vi "修改探头名称.vi"(9 "探头信息":string[](array[string]), 10 "原名称":string, 11 "输入信息":string) -> (0 "确定修改？":bool, 3 "新名称 o":string caption="新备注")   [LabVIEW 2017]
uses:
  <vilib>/addons/database/NI_Database_API.lvlib
panel:
  out "非空提示":string caption="字符串"
  in  "新名称":string caption="新备注"
  in  "取消":bool
  in  "确定":bool caption="OK2"
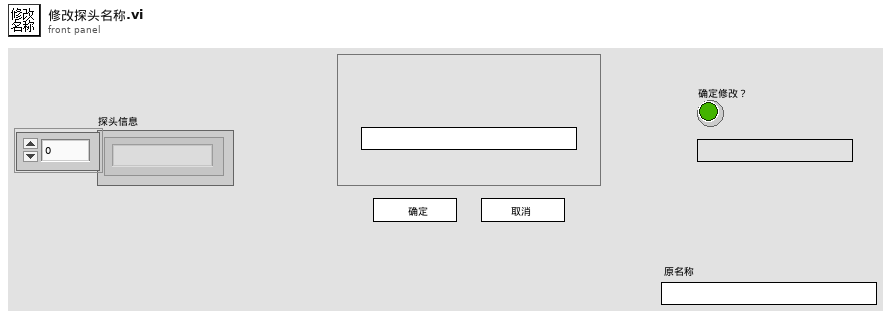
[diagram p1: front panel]
types:
  T1 = enum32{"Invalid", "Standard", "Closed", "Hidden", "Minimized", "Maximized"}
  T2 = cluster{"设备名称":string, "启用累积？":bool, "起始时间":timestamp, "累积剂量":dbl, "累积报警阈值":dbl}
  T3 = typedef "NI_Database_API.lvlib/Conn ObjectReference.ctl" = refnum<k1>
  T4 = cluster{"设备名称":string, "启用累积？":bool, "起始时间":timestamp, "累积剂量":dbl, "累积报警阈值":dbl}[]
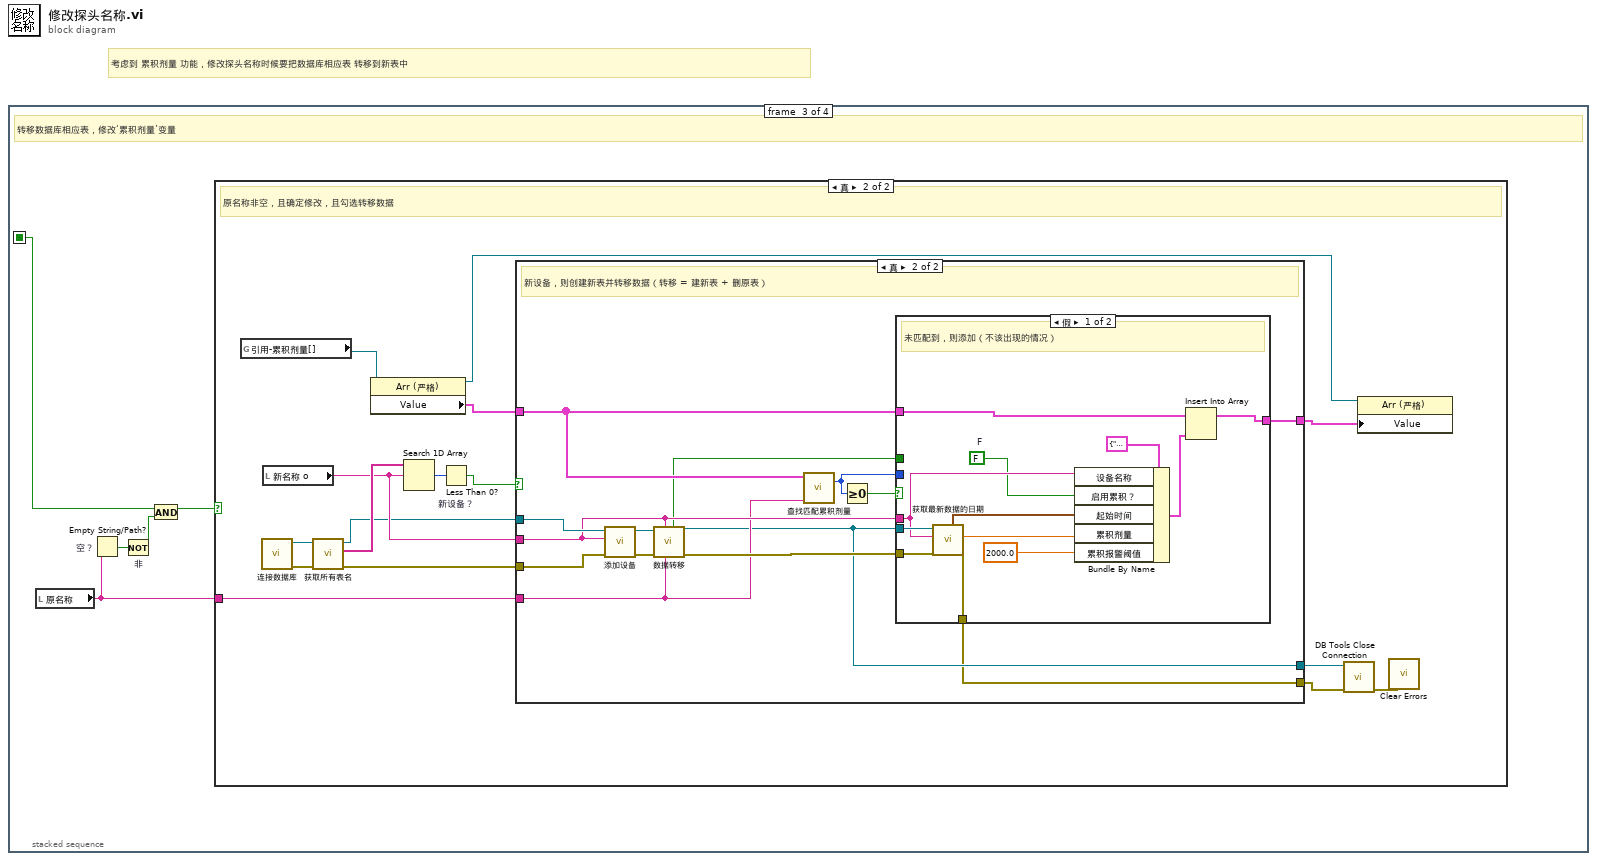
[diagram p0: block diagram]
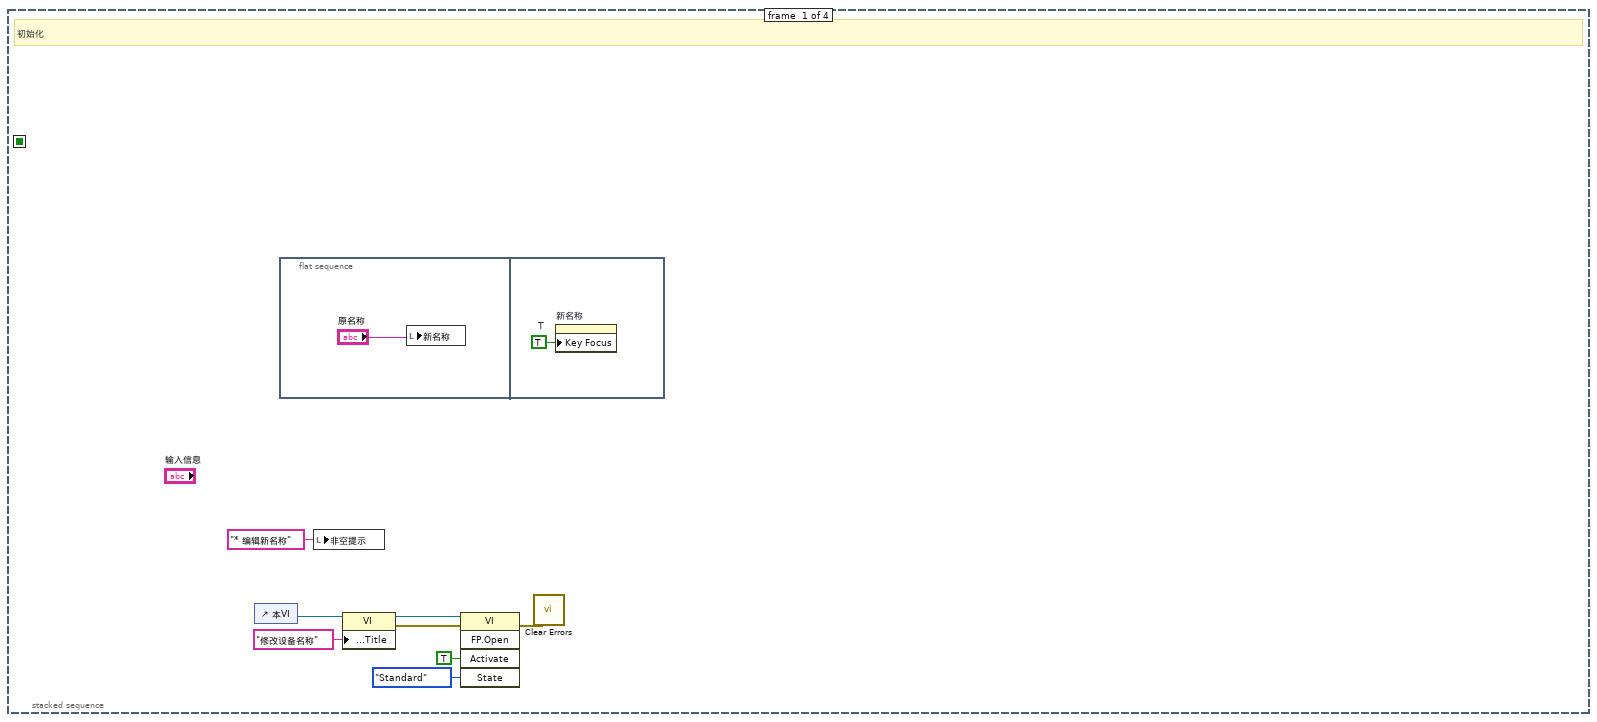
[diagram p2: hidden frame]
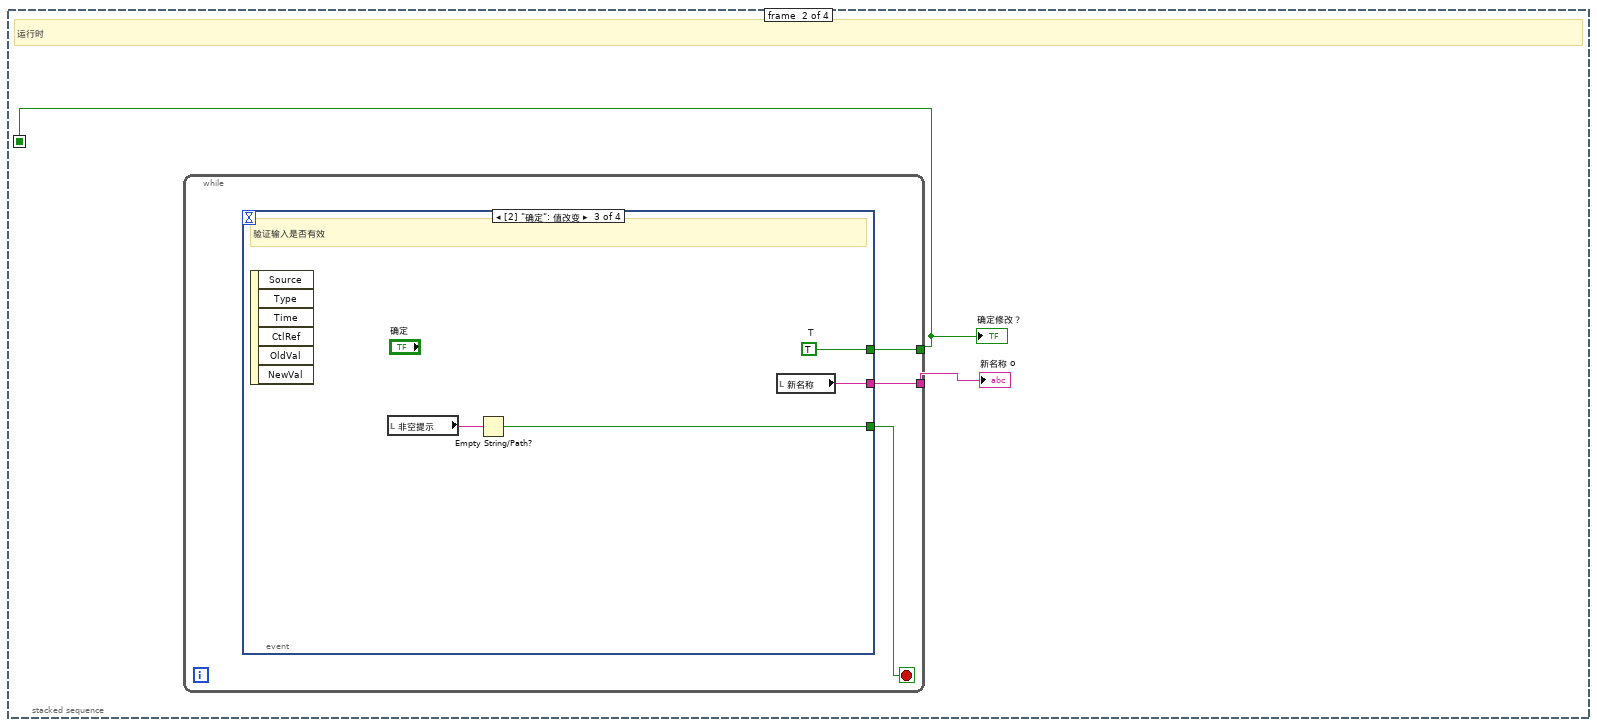
[diagram p3: hidden frame]
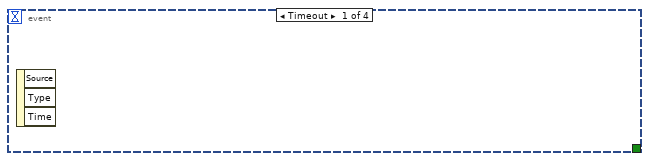
[diagram p4: hidden frame]
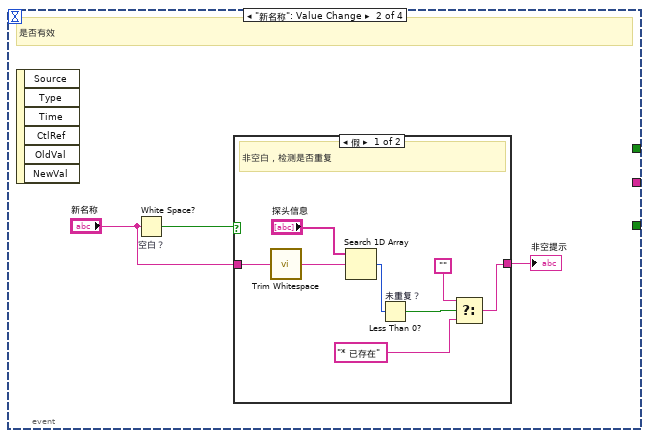
[diagram p5: hidden frame]
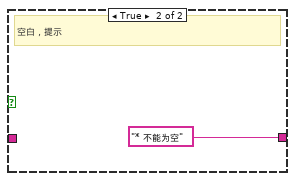
[diagram p6: hidden frame]
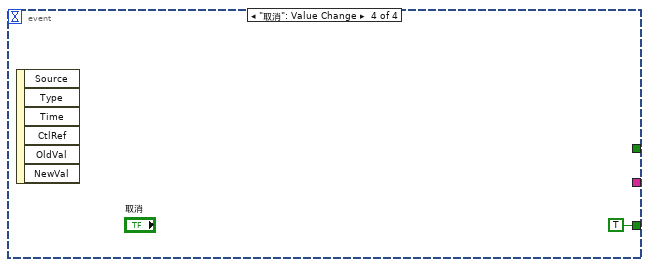
[diagram p7: hidden frame]
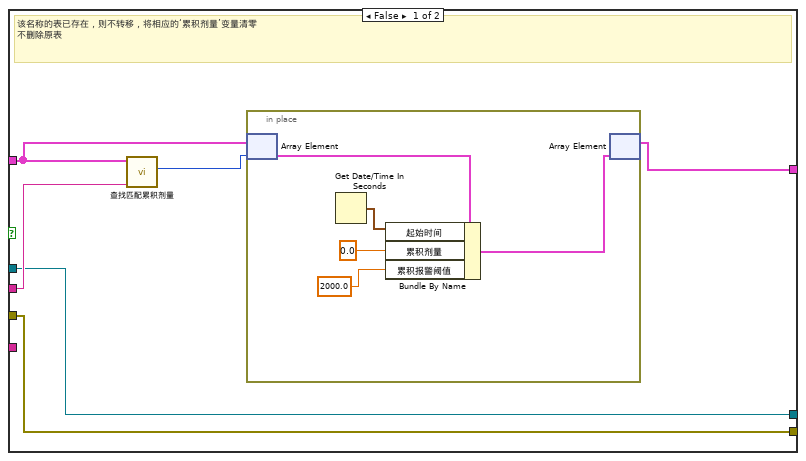
[diagram p9: hidden frame]
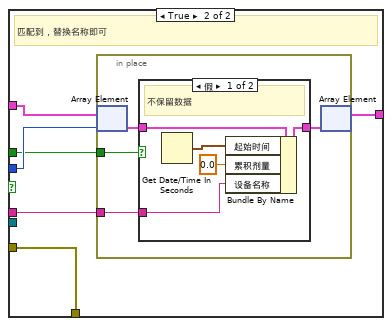
[diagram p10: hidden frame]
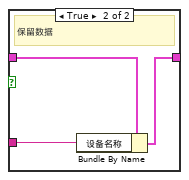
[diagram p11: hidden frame]
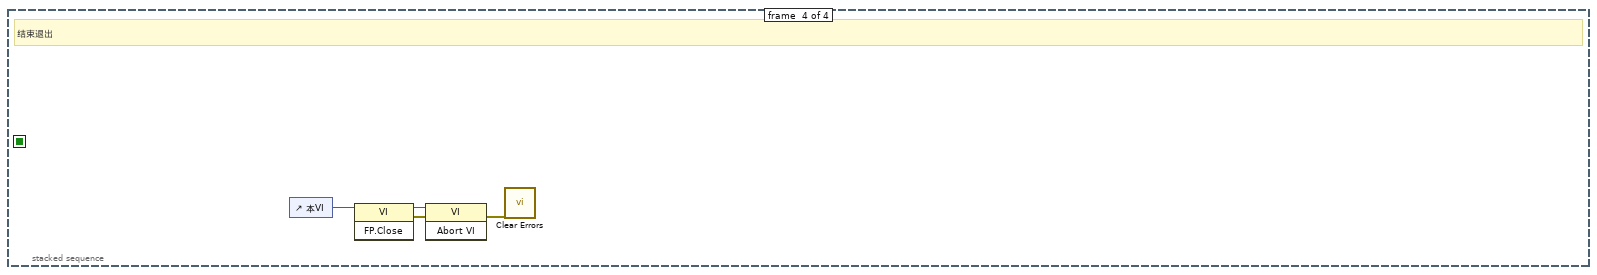
[diagram p12: hidden frame]
diagram:
  # "考虑到 累积剂量 功能，修改探头名称时候要把数据库相应表 转移到新表中"
  n1 = stacked-sequence {
    seq-local: [_ w11 _ _] -> [_ _ w37 _]
    frame #0 {
      # "初始化"
      n2 = control-ref of="本VI"() -> (w6:refnum<vi>)
      n3 = flat-sequence {
        frame #0 {
          n4 = local write "新名称"("原名称") -> ()
        }
        frame #1 {
          w10 = TRUE  # T
          n5 = property on="新名称" class="Str"("Key Focus"=w10) -> ()  [unwired: 2 in, 2 out]
        }
      }
      n6 = local write "非空提示"("* 编辑新名称" ("非空提示")) -> ()
      n7 = property class="VI"(reference=w6, "Front Panel.Title"="修改设备名称" ("前面板窗口:标题")) -> (reference out=w5:refnum<vi>, error out=w2:errorcluster)  [unwired: 1 in]
      n8 = invoke class="VI" method="FP.Open"(reference=w5, error in=w2, "Activate"=TRUE ("激活？"), "State"=T1."Standard" ("状态")) -> (error out=w1:errorcluster)  [unwired: 1 in, 4 out]
      n9 = call <vilib>:"Clear Errors.vi"("error in (no error)"=w1) -> ()  [unwired: 5 in, 2 out]
    }
    frame #1 {
      # "运行时"
      n10 = while {
        tunnel: [w14] -> w11
        tunnel: [w13] -> w12
        stop <- w15 stop-if-true
        n11 = event shown="[2] \"确定\": 值改变" {
          selector: _ -> [_ _ _ _]
          dyn-events: _ -> [_ _ _ _]
          timeout: _ -> [_ _ _ _]
          tunnel: [_ _ w30 TRUE] -> w15
          tunnel: [_ _ w29 _] -> w14
          tunnel: [_ _ w28 _] -> w13
          event Timeout {
            n12 = event-data() -> ()  [unwired: 1 in, 3 out]
          }
          event "新名称": Value Change {
            # "是否有效"
            n13 = event-data() -> ()  [unwired: 1 in, 6 out]
            n14 = White Space? "空白？"(1:"新名称") -> (0:w18:bool)
            n15 = case shown="假" w18 {
              tunnel: [w19 "* 不能为空" ("非空提示")] -> w17
              tunnel: "新名称" -> [w25 _]
              frame False {
                # "非空白，检测是否重复"
                n16 = call <vilib>:"Trim Whitespace.vi"("string"=w25) -> ("trimmed string"=w24:string)  [unwired: 1 in]
                n17 = Search 1D Array(1D array="探头信息", element=w24) -> (index of element=w23:i32)  [unwired: 1 in]
                n18 = Less Than 0? "未重复？"(x=w23) -> (x < 0?=w22:bool)
                n19 = Select(t="", s=w22, f="* 已存在") -> (s? t:f=w19:string)
              }
              frame True {
                # "空白，提示"
              }
            }
            "非空提示" <- w17
          }
          event "确定": Value Change {
            w29 = TRUE  # T
            # "验证输入是否有效"
            n20 = event-data() -> ()  [unwired: 1 in, 6 out]
            n21 = local read "非空提示"() -> (w31:string)
            n22 = Empty String/Path?(string/path=w31) -> (empty?=w30:bool)
            n23 = local read "新名称"() -> (w28:string)
          }
          event "取消": Value Change {
            n24 = event-data() -> ()  [unwired: 1 in, 6 out]
          }
        }
      }
      "新名称 o" <- w12
      "确定修改？" <- w11
    }
    frame #2 {
      # "转移数据库相应表，修改‘累积剂量’变量"
      n25 = local read "原名称"() -> (w36:string)
      n26 = Empty String/Path? "空？"(string/path=w36) -> (empty?=w35:bool)
      n27 = Not "非"(x=w35) -> (.not. x?=w33:bool)
      n28 = And(x=w37, y=w33) -> (x .and. y?=w34:bool)
      n29 = case shown="真" w34 {
        tunnel: w36 -> [_ w41]
        frame False {
          # "取消修改"
        }
        frame True {
          # "原名称非空，且确定修改，且勾选转移数据"
          n30 = global read "全局变量-35点监测.vi" "引用-累积剂量[]"() -> (w45:refnum<vi>)
          n31 = call "连接数据库.vi"() -> ("error out"=w53:errorcluster, "connection reference"=w52:T3)  [unwired: 10 in]
          n32 = local read "新名称 o"() -> (w48:string)
          n33 = call "获取所有表名.vi"("error in (no error)"=w53, "数据库连接引用 i"=w52) -> ("error out"=w47:errorcluster, "表名"=w51:string[], "数据库连接引用 o"=w46:T3)  [unwired: 7 in]
          n34 = property class="Arr (严格)"(reference=w45) -> (reference out=w43:refnum<vi>, "Value"=w44:T4)  [unwired: 1 in, 1 out]
          n35 = Search 1D Array(1D array=w51, element=w48) -> (index of element=w50:i32)  [unwired: 1 in]
          n36 = Less Than 0? "新设备？"(x=w50) -> (x < 0?=w49:bool)
          n37 = case shown="真" w49 {
            tunnel: w48 -> [w59 w72]
            tunnel: w47 -> [w54 w76]
            tunnel: w46 -> [w55 w75]
            tunnel: [w56 w71] -> w42
            tunnel: w41 -> [_ w69]
            tunnel: w44 -> [w58 w68]
            tunnel: [w55 w67] -> w40
            tunnel: [w54 w66] -> w39
            frame False {
              # "该名称的表已存在，则不转移，将相应的‘累积剂量’变量清零\n不删除原表"
              n38 = call "查找匹配累积剂量.vi"("探头名称"=w59, "累积剂量"=w58) -> ("匹配索引"=w57:i32)  [unwired: 7 in, 2 out]
              n39 = in-place {
                n40 = in-place-array #1(w58, w57) -> (w64:T2)
                n41 = Get Date/Time In Seconds() -> (seconds since 1Jan1904=w62:timestamp)
                n42 = Bundle By Name(cluster=w64, "起始时间"=w62, "累积剂量"=0.0, "累积报警阈值"=2000.0 ("累积剂量")) -> (w63:T2)
                n43 = in-place-array #1(w63) -> (w56:T4)  [unwired: 1 out]
              }
            }
            frame True {
              # "新设备，则创建新表并转移数据（转移 = 建新表 + 删原表）"
              n44 = call "添加设备.vi"("error in (no error)"=w76, "设备名称"=w72, "数据库连接引用 i"=w75) -> ("error out"=w77:errorcluster, "数据库连接引用 o"=w78:T3)  [unwired: 7 in]
              n45 = call "数据转移.vi"("原表名"=w69, "新表名"=w72, "error in (no error)"=w77, "数据库连接引用 i"=w78) -> ("error out"=w70:errorcluster, "数据库连接引用 o"=w67:T3, "保留数据？"=w65:bool)  [unwired: 5 in]
              n46 = call "查找匹配累积剂量.vi"("探头名称"=w69, "累积剂量"=w68) -> ("匹配索引"=w73:i32)  [unwired: 7 in, 2 out]
              n47 = Greater Or Equal To 0?(x=w73) -> (x >= 0?=w74:bool)
              n48 = case shown="假" w74 {
                tunnel: w73 -> [_ w95]
                tunnel: w68 -> [w88 w96]
                tunnel: w72 -> [w86 w94]
                tunnel: [w80 w93] -> w71
                tunnel: w67 -> [w90 _]
                tunnel: w70 -> [w89 w92]
                tunnel: [w79 w92] -> w66
                tunnel: w65 -> [_ w91]
                frame False {
                  w85 = FALSE  # F
                  # "未匹配到，则添加（不该出现的情况）"
                  n49 = call "获取最新数据的日期.vi"("error in (no error)"=w89, "表名"=w86, "数据库连接引用 i"=w90) -> ("error out"=w79:errorcluster, "累积值"=w83:dbl, "起始时间"=w84:timestamp)  [unwired: 4 in, 2 out]
                  n50 = Bundle By Name(cluster=T2 {"设备名称"="", "启用累积？"=FALSE, "起始时间"=timestamp(0 s since 1904-01-01), "累积剂量"=0.0, "累积报警阈值"=0.0} ("累积剂量"), "设备名称"=w86, "启用累积？"=w85, "起始时间"=w84, "累积剂量"=w83, "累积报警阈值"=2000.0) -> (w81:T2)
                  n51 = Insert Into Array(array=w88, new element=w81) -> (w80:T4)  [unwired: 1 in]
                }
                frame True {
                  # "匹配到，替换名称即可"
                  n52 = in-place {
                    in-place-border: w94 -> [w99]
                    in-place-border: w91 -> [w97]
                    n53 = in-place-array #2(w96, w95) -> (w100:T2)
                    n54 = case shown="假" w97 {
                      tunnel: w100 -> [w105 w108]
                      tunnel: w99 -> [w101 w107]
                      tunnel: [w104 w106] -> w98
                      frame False {
                        # "不保留数据"
                        n55 = Get Date/Time In Seconds() -> (seconds since 1Jan1904=w103:timestamp)
                        n56 = Bundle By Name(cluster=w105, "起始时间"=w103, "累积剂量"=0.0, "设备名称"=w101) -> (w104:T2)
                      }
                      frame True {
                        # "保留数据"
                        n57 = Bundle By Name(cluster=w108, "设备名称"=w107) -> (w106:T2)
                      }
                    }
                    n58 = in-place-array #2(w98) -> (w93:T4)  [unwired: 1 out]
                  }
                }
              }
            }
          }
          n59 = call <vilib>:"DB Tools Close Connection.vi"("error in (no error)"=w39, "connection reference"=w40) -> ("error out"=w38:errorcluster)  [unwired: 5 in]
          n60 = property class="Arr (严格)"(reference=w43, "Value"=w42) -> ()  [unwired: 1 in, 2 out]
          n61 = call <vilib>:"Clear Errors.vi"("error in (no error)"=w38) -> ()  [unwired: 5 in, 2 out]
        }
      }
    }
    frame #3 {
      # "结束退出"
      n62 = control-ref of="本VI"() -> (w112:refnum<vi>)
      n63 = invoke class="VI" method="FP.Close"(reference=w112) -> (reference out=w111:refnum<vi>, error out=w110:errorcluster)  [unwired: 2 in, 1 out]
      n64 = invoke class="VI" method="Abort VI"(reference=w111, error in=w110) -> (error out=w109:errorcluster)  [unwired: 1 in, 2 out]
      n65 = call <vilib>:"Clear Errors.vi"("error in (no error)"=w109) -> ()  [unwired: 5 in, 2 out]
    }
  }
